vi "Seq_SingleStep.vi"(8 "error in (no error)":errorcluster, 11 "Qbus in":refnum<class "Qbus.lvclass">) -> (0 "error out":errorcluster)   [LabVIEW 2016, in "SeqProcessor.lvlib"]
uses:
  SeqProcessor.lvlib
  <vilib>/addons/Qbus/Qbus.lvclass
  controls/Flag.ctl
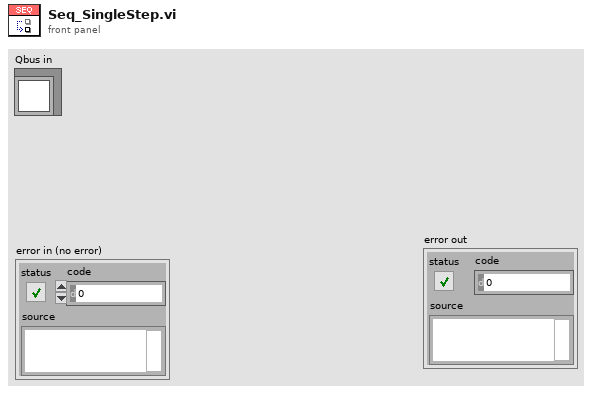
[diagram p1: front panel]
types:
  T1 = typedef "SeqProcessor.lvlib/Flag.ctl" = cluster{"SingleStep":bool, "Pause":bool, "Stop":bool, "StepbyStep":bool}
  T2 = typedef "SeqProcessor.lvlib/StepIndex.ctl" = cluster{"Index1":u32, "Index2":u32}
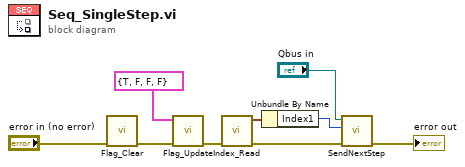
[diagram p0: block diagram]
diagram:
  n1 = call "Flag_Clear.vi"("error in (no error)"="error in (no error)") -> ("error out"=w3:errorcluster)  [unwired: 10 in]
  n2 = call "Flag_Update.vi"("error in (no error)"=w3, "Flag"=T1 {"SingleStep"=TRUE, "Pause"=FALSE, "Stop"=FALSE, "StepbyStep"=FALSE}) -> ("error out"=w2:errorcluster)  [unwired: 9 in]
  n3 = call "Index_Read.vi"("error in (no error)"=w2) -> ("error out"=w1:errorcluster, "Index"=w8:T2)  [unwired: 8 in, 1 out]
  n4 = Unbundle By Name(w8) -> ("Index1"=w6:u32)
  n5 = call "SendNextStep.vi"("error in (no error)"=w1, "StepIndex"=w6, "Qbus in"="Qbus in") -> ("error out"=→"error out":errorcluster)  [unwired: 8 in]
